vi "TCP Transmission Loop.vi"(11 "output cluster":T1) -> ()   [LabVIEW 2016]
uses:
  TCP Port Control.ctl
panel:
  out "Array":bool[](array[boolean])
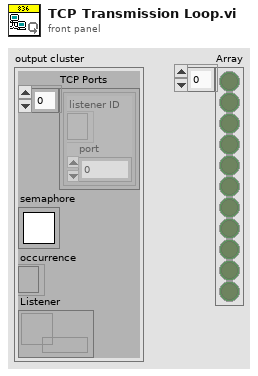
[diagram p1: front panel]
types:
  T1 = typedef "TCP Port Control.ctl" = cluster{"TCP Ports":cluster{"listener ID":refnum<k5>, "port":u16}[], "semaphore":T2, "occurrence":refnum<k4>, "Listener":refnum<data-value>}
  T2 = typedef "Semaphore RefNum" = refnum<k1>
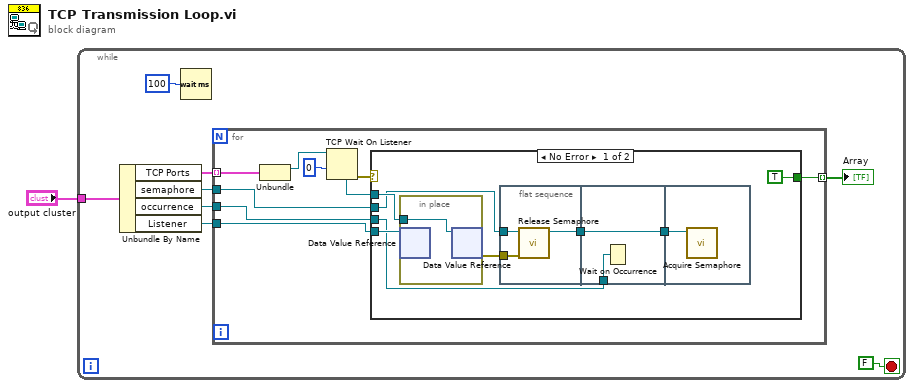
[diagram p0: block diagram]
diagram:
  n1 = while {
    tunnel: "output cluster" -> [w2]
    stop <- FALSE stop-if-true
    n2 = Unbundle By Name(w2) -> ("TCP Ports"=w6:cluster{"listener ID":refnum<k5>, "port":u16}[], "semaphore"=w3:T2, "occurrence"=w4:refnum<k4>, "Listener"=w5:refnum<data-value>)
    n3 = Wait (ms)(milliseconds to wait=u32 100) -> ()  [unwired: 1 out]
    n4 = for {
      tunnel: w6 -> [w14] mode=indexing
      tunnel: [w16] -> w8 mode=indexing
      tunnel: w3 -> [w13]
      tunnel: w5 -> [w12]
      tunnel: w4 -> [w11]
      n5 = Unbundle(w14) -> ("listener ID"=w15:refnum<k5>)  [unwired: 1 out]
      n6 = TCP Wait On Listener(9:0 ("timeout ms (wait forever: -1)"), 11:w15) -> (0:w17:errorcluster, 4:w10:refnum<k5>)  [unwired: 2 in, 3 out]
      n7 = case shown="No Error" w17 {
        tunnel: [TRUE _] -> w16
        tunnel: w13 -> [w22 _]
        tunnel: w10 -> [w24 _]
        tunnel: w12 -> [w25 _]
        tunnel: w11 -> [w23 _]
        frame No Error {
          n8 = in-place {
            in-place-border: w24 -> [w33]
            n9 = in-place-dvr #1(w25) -> ()  [unwired: 2 out]
            n10 = in-place-dvr #1(w33) -> (w21:errorcluster)  [unwired: 1 out]
          }
          n11 = flat-sequence {
            tunnel: w22 -> [w29]
            tunnel: w21 -> [w28]
            tunnel: [w27] -> w19
            tunnel: w23 -> [w31]
            tunnel: [w30] -> w20
            tunnel: w19 -> [w30]
            tunnel: w20 -> [w32]
            frame #0 {
              n12 = call <vilib>:"Release Semaphore.vi"("error in (no error)"=w28, "semaphore"=w29) -> ("semaphore out"=w27:T2)  [unwired: 4 in, 1 out]
            }
            frame #1 {
              n13 = Wait on Occurrence(2:w31) -> ()  [unwired: 2 in, 1 out]
            }
            frame #2 {
              n14 = call <vilib>:"Acquire Semaphore.vi"("semaphore"=w32) -> ()  [unwired: 4 in, 3 out]
            }
          }
        }
        frame Error {
        }
      }
    }
    "Array" <- w8
  }
